vi "svx_Polar_Convert_CustomizedMarkers.vi"(10 "polar plot":T3, 11 "customized marker":T1) -> (3 "customized annotations":T2)   [LabVIEW 2017, in "SVX Polar Plot.xctl"]
uses:
  <vilib>/addons/_XControls/Polar Plot/SVX Polar Plot.xctl
  <vilib>/Utility/miscctls.llb/LVAnnotationListTypeDef.ctl
  <vilib>/addons/_XControls/Polar Plot/subVIs/svx_Polar_Customized_Markers.ctl
  <vilib>/Analysis/NI_AALPro.lvlib
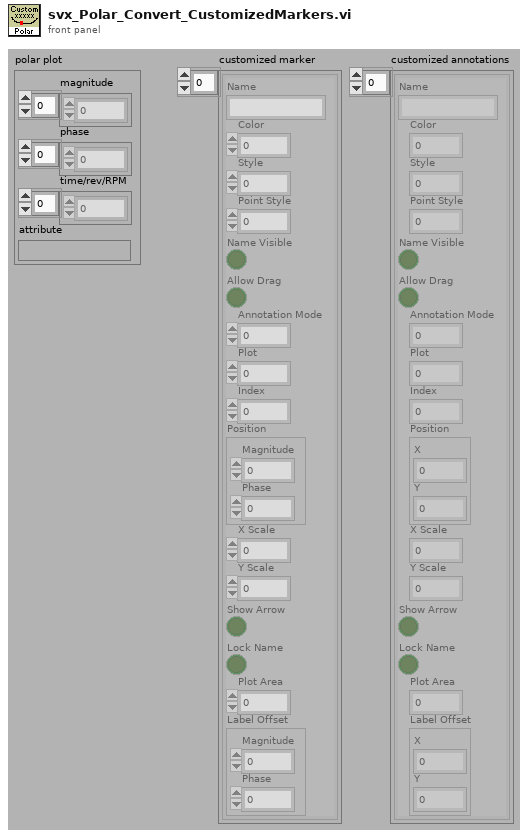
[diagram p1: front panel]
types:
  T1 = typedef "SVX Polar Plot.xctl/svx_Polar_Customized_Markers.ctl" = cluster{"Name":string, "Color":u32, "Style":u8, "Point Style":u8, "Name Visible":bool, "Allow Drag":bool, "Annotation Mode":u32, "Plot":i32, "Index":i32, "Position":cluster{"Magnitude":dbl, "Phase":dbl}, "X Scale":u32, "Y Scale":u32, "Show Arrow":bool, "Lock Name":bool, "Plot Area":i32, "Label Offset":cluster{"Magnitude":dbl, "Phase":dbl}}[]
  T2 = typedef "LVAnnotationListTypeDef.ctl" = cluster{"Name":string, "Color":u32, "Style":u8, "Point Style":u8, "Name Visible":bool, "Allow Drag":bool, "Annotation Mode":u32, "Plot":i32, "Index":i32, "Position":cluster{"X":dbl, "Y":dbl}, "X Scale":u32, "Y Scale":u32, "Show Arrow":bool, "Lock Name":bool, "Plot Area":i32, "Label Offset":cluster{"X":dbl, "Y":dbl}}[]
  T3 = cluster{"magnitude":dbl[], "phase":dbl[], "time/rev/RPM":dbl[], "attribute":variant}
  T4 = cluster{"Name":string, "Color":u32, "Style":u8, "Point Style":u8, "Name Visible":bool, "Allow Drag":bool, "Annotation Mode":u32, "Plot":i32, "Index":i32, "Position":cluster{"Magnitude":dbl, "Phase":dbl}, "X Scale":u32, "Y Scale":u32, "Show Arrow":bool, "Lock Name":bool, "Plot Area":i32, "Label Offset":cluster{"Magnitude":dbl, "Phase":dbl}}
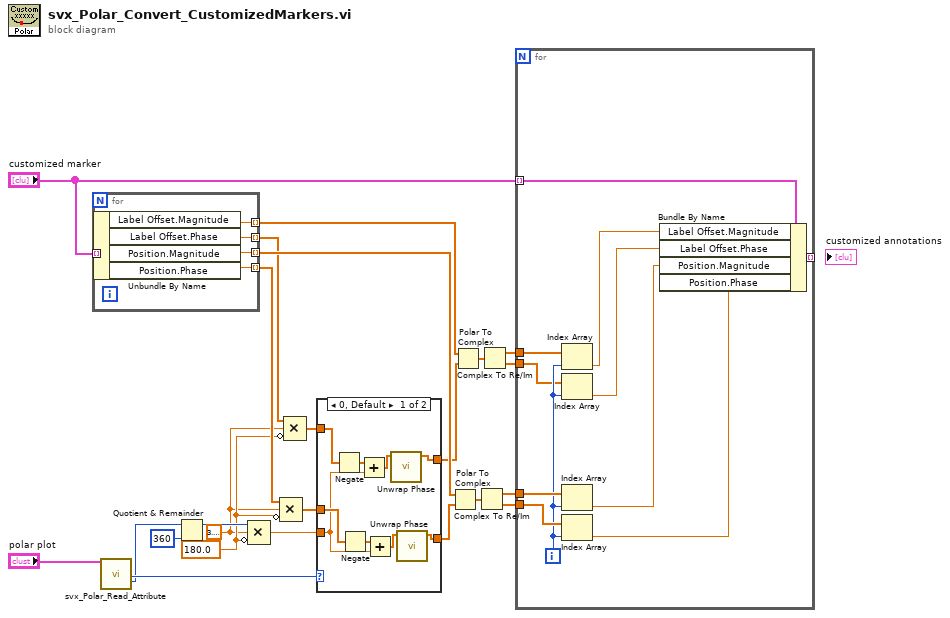
[diagram p0: block diagram]
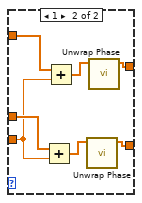
[diagram p2: hidden frame]
diagram:
  w10 = 180.0 ("value")
  w9 = 3.141592653589793
  n1 = for {
    tunnel: "customized marker" -> [w28] mode=indexing
    tunnel: [w27] -> w11 mode=indexing
    tunnel: [w26] -> w14 mode=indexing
    tunnel: [w25] -> w8 mode=indexing
    tunnel: [w24] -> w5 mode=indexing
    n2 = Unbundle By Name(w28) -> ("Label Offset.Magnitude"=w24:dbl, "Label Offset.Phase"=w25:dbl, "Position.Magnitude"=w27:dbl, "Position.Phase"=w26:dbl)
  }
  n3 = call <vilib>:"svx_Polar_Read_Attribute.vi"("polar plot"="polar plot") -> ("shaft rotating direction"=w17:u16, "probe angle [deg]"=w16:u16)  [unwired: 13 in, 4 out]
  n4 = Quotient & Remainder(x=w16, y=u16 360) -> (x-y*floor(x/y)=w22:u16)  [unwired: 1 out]
  n5 = Compound Arithmetic op=MULTIPLY(w22, w9, invert w10) -> (w20:dbl)
  n6 = Compound Arithmetic op=MULTIPLY(w14, w9, invert w10) -> (w18:dbl[])
  n7 = Compound Arithmetic op=MULTIPLY(w8, w9, invert w10) -> (w7:dbl[])
  n8 = case shown="0, Default" w17 {
    tunnel: w20 -> [w29 w39]
    tunnel: w18 -> [w35 w43]
    tunnel: [w36 w42] -> w19
    tunnel: w7 -> [w30 w40]
    tunnel: [w31 w38] -> w4
    frame 0, Default {
      n9 = Negate(x=w30) -> (-x=w33:dbl[])
      n10 = Negate(x=w35) -> (-x=w34:dbl[])
      n11 = Add(x=w33, y=w29) -> (x+y=w32:dbl[])
      n12 = Add(x=w34, y=w29) -> (x+y=w37:dbl[])
      n13 = call <vilib>:"Unwrap Phase.vi"("Phase"=w32) -> ("Unwrapped Phase"=w31:dbl[])  [unwired: 9 in, 1 out]
      n14 = call <vilib>:"Unwrap Phase.vi"("Phase"=w37) -> ("Unwrapped Phase"=w36:dbl[])  [unwired: 9 in, 1 out]
    }
    frame 1 {
      n15 = Add(x=w43, y=w39) -> (x+y=w44:dbl[])
      n16 = Add(x=w40, y=w39) -> (x+y=w41:dbl[])
      n17 = call <vilib>:"Unwrap Phase.vi"("Phase"=w44) -> ("Unwrapped Phase"=w42:dbl[])  [unwired: 9 in, 1 out]
      n18 = call <vilib>:"Unwrap Phase.vi"("Phase"=w41) -> ("Unwrapped Phase"=w38:dbl[])  [unwired: 9 in, 1 out]
    }
  }
  n19 = Polar To Complex(1:w19, 2:w11) -> (0:w23:cdb[])
  n20 = Polar To Complex(1:w4, 2:w5) -> (0:w6:cdb[])
  n21 = Complex To Re/Im(x + iy=w23) -> (x=w13:dbl[], y=w12:dbl[])
  n22 = Complex To Re/Im(x + iy=w6) -> (x=w3:dbl[], y=w2:dbl[])
  n23 = for {
    tunnel: "customized marker" -> [w50] mode=indexing
    tunnel: w13 -> [w55]
    tunnel: w12 -> [w54]
    tunnel: w3 -> [w52]
    tunnel: w2 -> [w51]
    tunnel: [w49] -> _ mode=indexing
    i -> [w53]
    n24 = Index Array(array=w52, index=w53) -> (element=w46:dbl)
    n25 = Index Array(array=w51, index=w53) -> (element=w45:dbl)
    n26 = Index Array(array=w55, index=w53) -> (element=w48:dbl)
    n27 = Index Array(array=w54, index=w53) -> (element=w47:dbl)
    n28 = Bundle By Name(cluster=w50, "Label Offset.Magnitude"=w46, "Label Offset.Phase"=w45, "Position.Magnitude"=w48, "Position.Phase"=w47) -> (w49:T4)
  }
